vi "Correct funct acq lengths.vi"(8 "error in (no error)":errorcluster, 11 "Cool-down time (s)":refnum<vi>) -> (0 "error out":errorcluster, 2 "Cool-down time (s)":dbl, 3 "Cool-down time (s)":refnum<vi>)   [LabVIEW 2020]
uses:
  Typedefs/ROI management FG states.ctl
  User Interface/ROI Entry screen/Globals/gl_ROI Entry UI globals.vi
  Global Variables/General Globals.vi
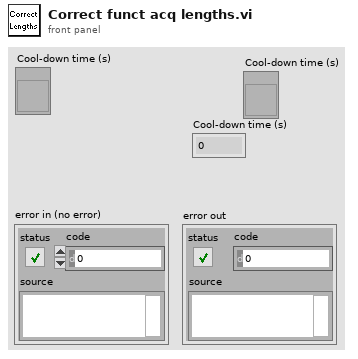
[diagram p1: front panel]
types:
  T1 = typedef "ROI management FG states.ctl" = enum16{"Read", "Write", "Write-from dataset", "Clear Last", "Clear All", "Delete ROI", "Update ROIs time", "Reload last ROI set", "Modify ROI Parameters", "Offset all ROI", "Offset visible ROI", "Modify Dwell Time", "Modify Laser Power"}
  T2 = typedef "ROI entry screen ctrl refs cluster.ctl" = cluster{"Done button":refnum<vi>, "Imaging button":refnum<vi>, "Acquisition button":refnum<vi>, "Scan dwell time per pixel (us)":refnum<vi>, "# of planes":refnum<vi>, "Zoom Ctrl":refnum<vi>, "Equal size":refnum<vi>, "Channel":refnum<vi>, "Image Display":refnum<vi>, "Z-Plane Selector":refnum<vi>, "Number of lines left":refnum<vi>, "Z-stack folder path":refnum<vi>, "POI Density":refnum<vi>, "Arb Plane Entry":refnum<vi>, "Whole Plane":refnum<vi>, "Line Mode":refnum<vi>, "Clear Last":refnum<vi>, "Clear All":refnum<vi>, "Delete Lines":refnum<vi>, "Trial Length (sec)":refnum<vi>, "Palette Type":refnum<vi>, "Intensity slider":refnum<vi>, "# POI":refnum<vi>, "Max Z Proj":refnum<vi>, "Zplane ind":refnum<vi>, "Wavelength (nm)":refnum<vi>, "Number of Trials":refnum<vi>, "Funct stim.trig.enable":refnum<vi>, "Funct stim.trig.delay (s)":refnum<vi>, "Line Mode":refnum<vi>, "Step size (µm)":refnum<vi>, "ROI move mode":refnum<vi>, "Cool-down time (s)":refnum<vi>, "Enable cool-down time":refnum<vi>, "Motor Z ind. (um)":refnum<vi>, "AOL Z ind. (um)":refnum<vi>, "Load Reference Image":refnum<vi>, "Rel.  Res.":refnum<vi>, "ROI LIST":refnum<vi>, "Show All":refnum<vi>, "ROI Type":refnum<vi>, "Start Plane":refnum<vi>, "Stop Plane":refnum<vi>, "Offset ROI":refnum<vi>, "Tab Control":refnum<vi>, "Laser Power(%)":refnum<vi>, "Cycle rate":refnum<vi>, "FOV (Ind.)":refnum<vi>, "Frame Size (Ind.)":refnum<vi>, "Resolution (Ind.)":refnum<vi>, "Pixel Density (Ind)":refnum<vi>, "Laser Power (Ind.)":refnum<vi>, "Dwell Time (Ind.)":refnum<vi>, "Adj MC":refnum<vi>}
  T3 = typedef "ROI parameters data type.ctl" = cluster{"ROI index":dbl, "ROI ID":dbl, "ROI Time (ns)":dbl, "Pixels in ROI":dbl, "X start":dbl, "Y start":dbl, "Z start":dbl, "X stop":dbl, "Y stop":dbl, "Z stop":dbl, "Angle (deg)":dbl, "Composite ID":dbl, "Number of lines":dbl, "Frame Size":dbl, "Zoom":dbl, "Laser Power (%)":dbl, "ROI group ID":dbl, "Resolution":dbl, "Dwell Time per pixel":dbl, "Pixels per miniscan":dbl, "Original FOV (um)":dbl, "Apparent Frame Size":dbl, "Z Plane Idx":i32[], "Z Plane codes":i32[]}
  T4 = typedef "AOL_Globals.ctl" = cluster{"Imaging Protocol":T5, "Number of POI":u16, "Number of Miniscans":u16, "Number of Trials":u16, "Number of Cycles ":u64, "# Averaged Frames":u16, "Laser power (%)":u8, "Pockels (V)":dbl, "Acquisition Length (sec)":dbl, "Fill time (us)":dbl, "POI Dwell time (us)":dbl, "Miniscan Dwell time per pixel (us)":dbl, "PMT 1":dbl, "PMT 2":dbl, "Back Apperture (mA)":dbl, "Frame Size":T6, "Center Frequency":dbl, "Field of View (norm)":dbl, "DwellTime (us)":dbl, "Wavelength (nm)":dbl, "Zoom":dbl, "AOL Z":dbl, "AOL Mode":T7, "GridXY":dbl, "GridZ":dbl, "TriggerPeriod (sec)":dbl, "Number of Pixels in Miniscan":u16, "Experiment folder path":path, "X centre":dbl, "Y centre":dbl, "Angle (degrees)":dbl, "Plane Mode":T8, "Threshold":u16[], "Regenerate Chirps":bool, "Rectangle ROI length (pixels)":u16, "Rectangle ROI height (pixels)":u16, "AOD fill":u16, "StartupDelay":i32, "Samples Wait after Trigger":u16, "Slip Cycle":u32, "Add Cycle":bool, "Functional Mode":T9, "Z Start":dbl, "Z Stop":dbl, "# Planes":i32, "Total Pixels":i32, "Variable Miniscan Pixels":u16[], "Use Variable Length":bool, "Use Variable Resolution":bool, "Laser power (%) at Z Start":u8, "Laser power (%) at Z Stop":u8, "Ref Z Step":i8, "Ref Dwell Time (us)":dbl, "Field of View (um)":dbl}
  T5 = typedef "Imaging Protocols enum.ctl" = enum16{"AOL Z-Stack", "Motor Z Stack", "Functional Acquisition", "Single Plane Acquisition", "Volume Acquisition", "Live Imaging", "Live Plane Imaging", "Live Volume Imaging"}
  T6 = typedef "Frame Size.ctl" = u16
  T7 = typedef "AOL modes.ctl" = enum16{"Raster", "Structural", "Pointing", "Mini Scan", "Alignment"}
  T8 = typedef "Plane Mode.ctl" = u16
  T9 = typedef "Functional Mode.ctl" = enum16{"Point", "Line", "Patch", "Plane", "Volume"}
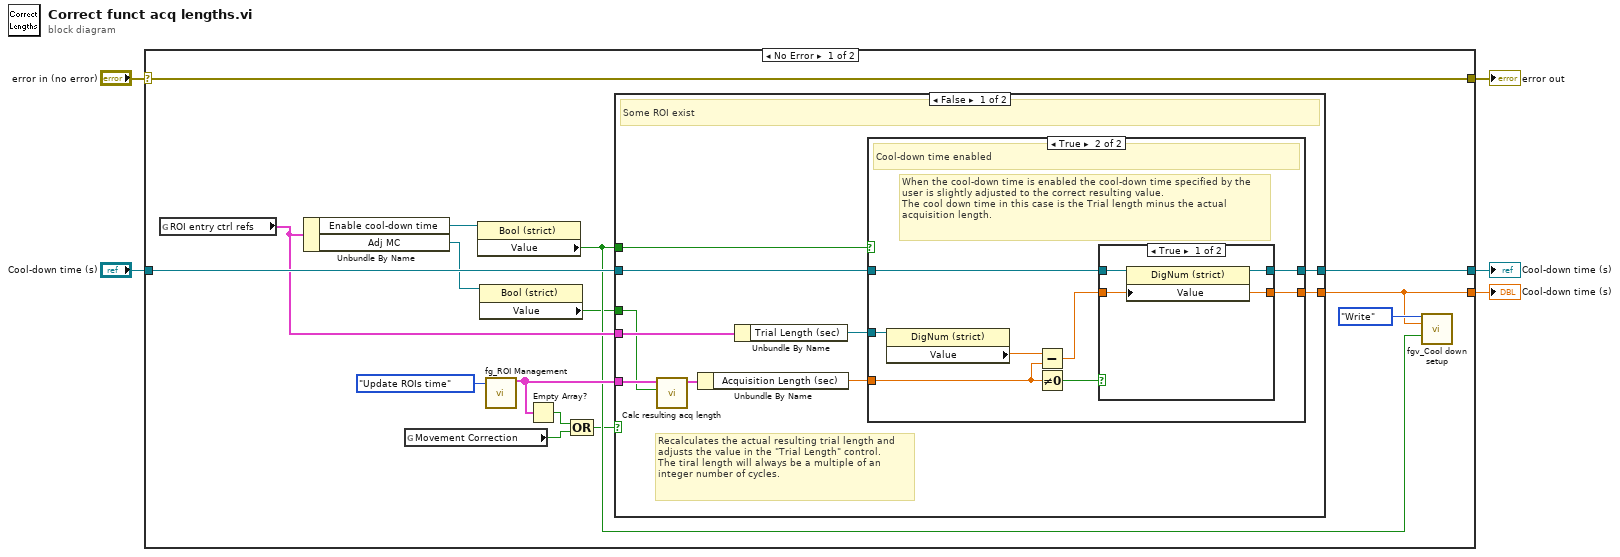
[diagram p0: block diagram]
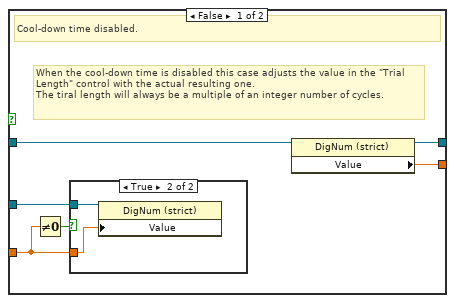
[diagram p2: hidden frame]
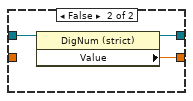
[diagram p4: hidden frame]
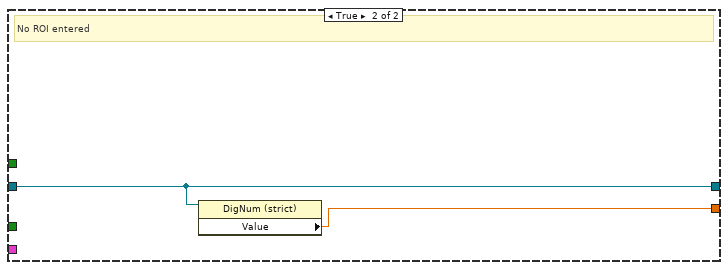
[diagram p5: hidden frame]
diagram:
  n1 = case shown="No Error" "error in (no error)" {
    selector: "error in (no error)" -> [w18 w56]
    tunnel: [w18 w56] -> w5
    tunnel: "Cool-down time (s)" -> [w20 w55]
    tunnel: [w14 _] -> w2
    tunnel: [w19 w55] -> w1
    frame No Error {
      n2 = global read "gl_ROI Entry UI globals.vi" "ROI entry ctrl refs"() -> (w12:T2)
      n3 = Unbundle By Name(w12) -> ("Enable cool-down time"=w13:refnum<vi>, "Adj MC"=w7:refnum<vi>)
      n4 = global read "General Globals.vi" "Movement Correction"() -> (w10:bool)
      n5 = property on="Property Node" class="Bool (strict)"(reference=w13) -> ("Value"=w11:bool)  [unwired: 1 in, 2 out]
      n6 = property on="Property Node" class="Bool (strict)"(reference=w7) -> ("Value"=w6:bool)  [unwired: 1 in, 2 out]
      n7 = call "fg_ROI Management.vi"("Function"=ROI_management_FG_states."Update ROIs time") -> ("ROI Setup"=w16:T3[])  [unwired: 8 in, 6 out]
      n8 = Empty Array?(array=w16) -> (empty?=w9:bool)
      n9 = Compound Arithmetic op=OR(w9, w10) -> (w8:bool)
      n10 = case shown="False" w8 {
        tunnel: w20 -> [w30 w54]
        tunnel: [w29 w53] -> w14
        tunnel: [w28 w54] -> w19
        tunnel: w16 -> [w27 _]
        tunnel: w11 -> [w23 _]
        tunnel: w12 -> [w22 _]
        tunnel: w6 -> [w21 _]
        frame False {
          # "Recalculates the actual resulting trial length and adjusts the value in the \"Trial Length\" control.\nThe tiral length will always be a multiple of an integer number of cycles."
          # "Some ROI exist"
          n11 = call "Calc resulting acq length.vi"("Adjust for MC ?"=w21, "XYZ_Coordinates"=w27) -> ("Output cluster"=w26:T4)  [unwired: 8 in, 1 out]
          n12 = Unbundle By Name(w26) -> ("Acquisition Length (sec)"=w25:dbl)
          n13 = Unbundle By Name(w22) -> ("Trial Length (sec)"=w24:refnum<vi>)
          n14 = case shown="True" w23 {
            tunnel: w30 -> [w34 w46]
            tunnel: [w35 w45] -> w28
            tunnel: [w33 w39] -> w29
            tunnel: w25 -> [w31 w41]
            tunnel: w24 -> [w36 w43]
            frame False {
              # "When the cool-down time is disabled this case adjusts the value in the \"Trial Length\" control with the actual resulting one.\nThe tiral length will always be a multiple of an integer number of cycles."
              # "Cool-down time disabled."
              n15 = Not Equal To 0?(x=w31) -> (x != 0?=w32:bool)
              n16 = case shown="True" w32 {
                tunnel: w31 -> [_ w38]
                tunnel: w36 -> [_ w37]
                frame False {
                }
                frame True {
                  n17 = property on="Property Node" class="DigNum (strict)"(reference=w37, "Value"=w38) -> ()  [unwired: 1 in, 2 out]
                }
              }
              n18 = property on="Property Node" class="DigNum (strict)"(reference=w34) -> (reference out=w35:refnum<vi>, "Value"=w33:dbl)  [unwired: 1 in, 1 out]
            }
            frame True {
              # "When the cool-down time is enabled the cool-down time specified by the user is slightly adjusted to the correct resulting value.\nThe cool down time in this case is the Trial length minus the actual acquisition length."
              # "Cool-down time enabled"
              n19 = property on="Property Node" class="DigNum (strict)"(reference=w43) -> ("Value"=w44:dbl)  [unwired: 1 in, 2 out]
              n20 = Subtract(x=w44, y=w41) -> (x-y=w42:dbl)
              n21 = Not Equal To 0?(x=w41) -> (x != 0?=w40:bool)
              n22 = case shown="True" w40 {
                tunnel: w46 -> [w49 w52]
                tunnel: [w48 w51] -> w45
                tunnel: w42 -> [w47 _]
                tunnel: [w47 w50] -> w39
                frame True {
                  n23 = property on="Property Node" class="DigNum (strict)"(reference=w49, "Value"=w47) -> (reference out=w48:refnum<vi>)  [unwired: 1 in, 1 out]
                }
                frame False {
                  n24 = property on="Property Node" class="DigNum (strict)"(reference=w52) -> (reference out=w51:refnum<vi>, "Value"=w50:dbl)  [unwired: 1 in, 1 out]
                }
              }
            }
          }
        }
        frame True {
          # "No ROI entered"
          n25 = property on="Property Node" class="DigNum (strict)"(reference=w54) -> ("Value"=w53:dbl)  [unwired: 1 in, 2 out]
        }
      }
      n26 = call "fgv_Cool down setup.vi"("Function"=enum16{"Intialize", "Write", "Read", "Clear"}."Write", "Cool-down time (s)"=w14, "Enable cool-down time"=w11) -> ()  [unwired: 10 in, 3 out]
    }
    frame Error {
    }
  }
  "error out" <- w5
  "Cool-down time (s)" <- w1
  "Cool-down time (s)" <- w2
